vi "Update Script Listbox.vi"(10 "standard output":string, 11 "ListBox in":refnum<vi>) -> ()   [LabVIEW 2023, in "Script.lvclass"]
uses:
  Script.lvclass
  Script.lvclass/Script.ctl
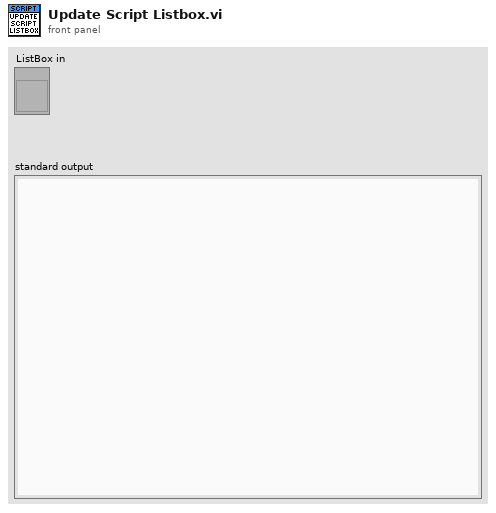
[diagram p1: front panel]
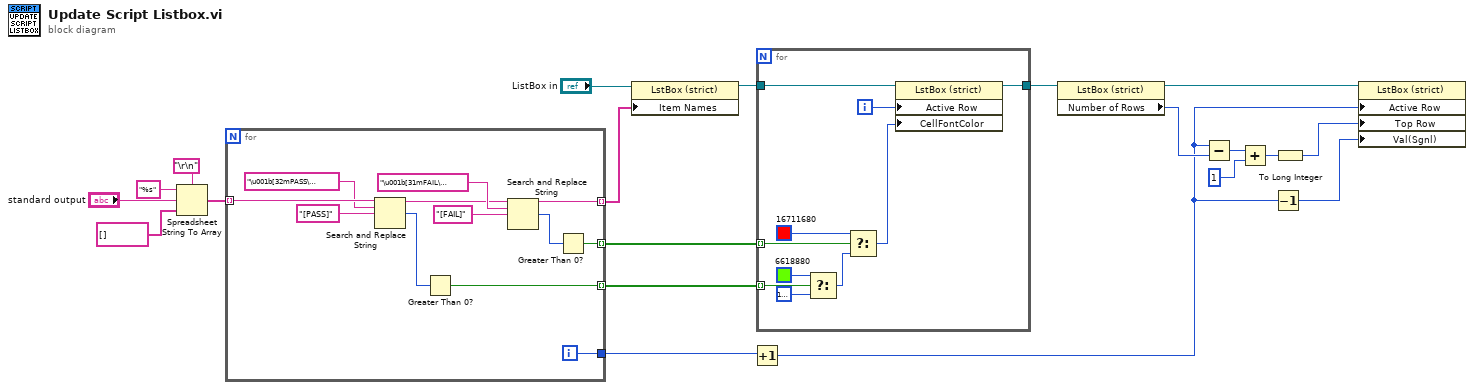
[diagram p0: block diagram]
diagram:
  n1 = Spreadsheet String To Array(delimiter (Tab)="\r\n", format string="%s", spreadsheet string="standard output", array type (2D Dbl)=string[] []) -> (array=w3:string[])
  n2 = for {
    tunnel: w3 -> [w32] mode=indexing
    tunnel: [w28] -> w10 mode=indexing
    tunnel: [w27] -> w8
    tunnel: [w22] -> w2 mode=indexing
    tunnel: [w21] -> w1 mode=indexing
    i -> [w27]
    n3 = Search and Replace String(input string=w32, search string="\u001b[32mPASS\u001b[0m", replace string="[PASS]" ("replace string (\"\")")) -> (result string=w23:string, number of replacements=w29:i32)  [unwired: 5 in, 2 out]
    n4 = Greater Than 0?(x=w29) -> (x > 0?=w28:bool)
    n5 = Search and Replace String(input string=w23, search string="\u001b[31mFAIL\u001b[0m", replace string="[FAIL]" ("replace string (\"\")")) -> (result string=w22:string, number of replacements=w26:i32)  [unwired: 5 in, 2 out]
    n6 = Greater Than 0?(x=w26) -> (x > 0?=w21:bool)
  }
  n7 = property class="LstBox (strict)"(reference="ListBox in", "Item Names"=w2) -> (reference out=w9:refnum<vi>)  [unwired: 1 in, 1 out]
  n8 = Increment(x=w8) -> (x+1=w5:i32)
  n9 = for {
    tunnel: w9 -> [w42]
    tunnel: w10 -> [w40] mode=indexing
    tunnel: [w38] -> w6
    tunnel: w1 -> [w36] mode=indexing
    i -> [w41]
    n10 = Select(t=u32 6618880, s=w40, f=u32 16777225) -> (s? t:f=w34:u32)
    n11 = Select(t=u32 16711680, s=w36, f=w34) -> (s? t:f=w33:u32)
    n12 = property class="LstBox (strict)"(reference=w42, "Active Row"=w41, "CellFontColor"=w33) -> (reference out=w38:refnum<vi>)  [unwired: 1 in, 1 out]
  }
  n13 = property class="LstBox (strict)"(reference=w6) -> (reference out=w4:refnum<vi>, "Number of Rows"=w7:u32)  [unwired: 1 in, 1 out]
  n14 = Subtract(x=w5, y=w7) -> (x-y=w16:u32)
  n15 = Add(x=w16, y=u32 1) -> (x+y=w18:u32)
  n16 = Decrement(x=w5) -> (x-1=w19:i32)
  n17 = To Long Integer(number=w18) -> (32bit integer=w11:i32)
  n18 = property class="LstBox (strict)"(reference=w4, "Active Row"=w5, "Top Row"=w11, "Val(Sgnl)"=w19) -> ()  [unwired: 1 in, 2 out]
